vi "Record in xml and EQdb.vi"(8 "error in":errorcluster, 11 "?":T1) -> (0 "error out":errorcluster, 1 "Database primary key":i32, 2 "Variant return data":variant, 3 "Serial number out":string)   [LabVIEW 2018]
uses:
  State data/Records.ctl
  <userlib>/nEQdb/Test Data classes/Basic Data/nEQdb data base enums.ctl
  <userlib>/nEQdb/Test Data classes/Basic Data/Basic Data.lvclass
  C:/Program Files (x86)/National Instruments/LabVIEW 2018/user.lib/nEQdb/Test Data classes/Test Data.lvclass
  <userlib>/nEQdb/Test Data classes/Test Data.lvclass
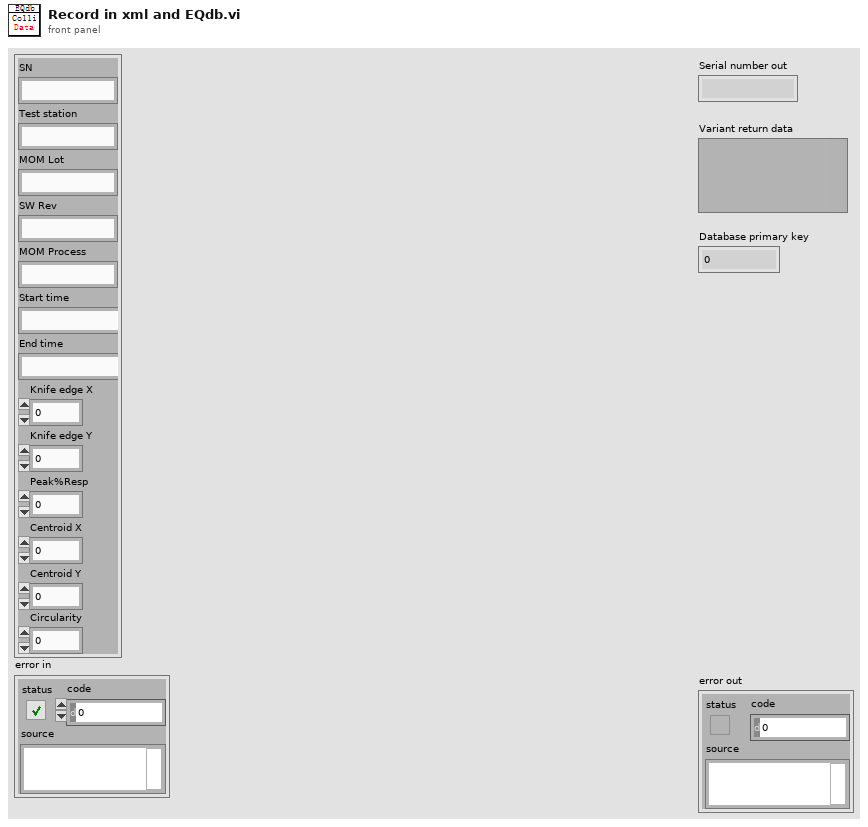
[diagram p1: front panel]
types:
  T1 = typedef "Records.ctl" = cluster{"SN":string, "Test station":string, "MOM Lot":string, "SW Rev":string, "MOM Process":string, "Start time":string, "End time":string, "Knife edge X":dbl, "Peak%Resp":dbl, "Centroid X":dbl, "Knife edge Y":dbl, "Centroid Y":dbl, "Circularity":dbl}
  T2 = typedef "Basic Data.lvclass/nEQdb data base enums.ctl" = enum16{"No enum selected", "Serial number 1", "Test number 2", "Subtest type 3", "Subtest number 4", "Datapoint 5", "Operator 6", "Water temperature supply 7", "Water temperature return 8", "Water pressure supply 9", "Water pressure return 10", "Water flow rate supply 11", "Water flow rate return 12", "Test parameter file 13", "Workorder number 14", "Workorder operation number 15", "Thermal resistance degcperw 16", "Thermal resistance mpera 17", "Current source model 18", "Current source sn 19", "Power meter model 20", "Power meter sn 21", "Power meter head model 22", "Power meter head sn 23", "Threshold current 24", "Slope efficiency 25", "Temperature set 26", "Temperature measured at test start 27", "Power auxilary units 28", "Power auxilary description 29", "Temporary auxilary description 30", "Itar 31", "Dynamic resistance 32", "Voltage intercept 33", "Calibration current 34", "Current set 35", "Current measured 36", "Optical power 37", "Voltage diode 38", "Voltage compliance 39", "Temperature measured 40", "Efficiency diode 41", "Voltage tec 42", "Current tec 43", "Detector responsivity 44", "Detector responsivity wavelength 45", "Power auxilary 46", "Temperature auxilary 47", "Start datetime 48", "End datetime 49", "Centroid 50", "Peak 51", "Fwhm 52", "Fw1 e 2m 53", "Fw1 e 3m 54", "Pulse width 55", "Prf 56", "Osa sensitivity 57", "Osa samples 58", "Osa resolution 59", "Osa averaging 60", "Test station 61", "Additional instruments model 62", "Additional instruments sn 63", "Osa model 64", "Osa sn 65", "Multi stage test key 66", "Good emitters 67", "Wavelength 68", "Intensity 69", "Position 70", "Operating power 71", "Schema 72", "Centroid as pixel 73", "Polarization 74", "Intensity te 75", "Intensity tm 76", "Intensity baseline 77", "Te ratio 78", "Current set scan 79", "Current measured scan 80", "Centroid temporal variation 81", "Voltage 82", "Current 83", "Volt meter model 84", "Volt meter sn 85", "Angle 86", "Farfield axis 87", "Item 88", "Activity 89", "Limit 90", "Operating power spec 91", "Operating current spec 92", "Operating voltage 93", "Operating efficiency 94", "Operating resistance 95", "Reverse bias leakage current 96", "Threshold current change 97", "Slope efficiency change 98", "Operating current change 99", "Active date 100", "Active notes 101", "Eco number 102", "Test notes 103", "Spectral map 104", "Test id from test station 105", "Is image 106", "Image pathname 107", "Datetime 108", "Grade initial 109", "Grade final 110", "Workorder operation name 111", "Engineering grading field 112", "Slope efficiency spec 113", "Threshold current spec 114", "Auxilary identifier 115", "Fwhm fa 116", "Telescope magnification 117", "Measurement lens focal length 118", "Te ratio spec 119", "Wavelength fwhm operating spec 120", "Wavelength fw1e2m operating spec 121", "Prebi slope efficiency spec 122", "Prebi operating current spec 123", "Controlled spec 124", "Wavelength centroid spec 125", "Divergence na 90  incl spec 126", "Wavelength temperature coefficient spec 127", "Operating temperature spec 128", "Fast axis divergence fw1e2m spec 129", "Slow axis divergence fw1e2m spec 130", "Rows of chiplets 131", "Columns of chiplets 132", "Divergence na 90  incl 133", "Fast axis divergence fwhm spec 134", "Slow axis divergence fwhm spec 135", "Farfield current 136", "Nearfield current 137", "Nearfield fwhm 138", "Nearfield fw1e2m 139", "Operating power validation spec 140", "Reverse bias leakage current validation spec 141", "Operating resistance validation spec 142", "Threshold current validation spec 143", "Threshold current change validation spec 144", "Slope efficiency validation spec 145", "Slope efficiency change validation spec 146", "Operating current validation spec 147", "Operating current change validation spec 148", "Te ratio validation spec 149", "Operating efficiency validation spec 150", "Operating voltage validation spec 151", "Thermal resistance degcperw validation spec 152", "Wavelength fwhm validation spec 153", "Wavelength fw1e2m validation spec 154", "Validation wavelength current validation spec 155", "Number of emitters validation spec 156", "Fast axis divergence fwhm validation spec 157", "Slow axis divergence fwhm validation spec 158", "External power supply voltage 159", "Bay 160", "Lens magnification 161", "Scan type 162", "Scan file 163", "Measured optical power 164", "Beam width short axis 165", "Beam length short axis 166", "Beam non uniformity 167", "Beam local non uniformity 168", "Total optical power 169", "Power density 170", "Relative beam position 171", "Subtesttype name 172", "Subtest name 173", "Laser number 174", "System temp label 175", "System flow label 176", "Ldd number 177", "Ldd laser number 178", "Additional instrument description 179", "Micrometer position 180", "Stage position x 181", "Stage position y 182", "Stage position z 183", "Stage position roll 184", "Stage position yaw 185", "Stage position pitch 186", "Mean maximum temperature 187", "Absolute pressure 60s after minimum 188", "Stage position align power 189", "Stage position number 190", "Stage position max align power 191", "Efficiency peak spec 192", "O to o spec 193", "Unit 194", "Qty per series 195", "Qty 196", "Used at operation number 197", "New or already released 198", "Route 199", "Itemname 200", "Recipe name 201", "Maskdatum1 x coord 202", "Maskdatum1 y coord 203", "Maskdatum2 x coord 204", "Maskdatum2 y coord 205", "Layer 206", "Emitter location file pathname 207", "Time 208", "Defect number 209", "X coord 210", "Y coord 211", "Classification 212", "Perimeter straightness 213", "Area width 214", "Brightness 215", "Area diameter 216", "Surface range 217", "Surface range x 218", "Surface range y 219", "Surface gradient 220", "Surface gradient x 221", "Surface gradient y 222", "Maximum gradient x 223", "Area gradient x 224", "Density gradient x 225", "Maximum gradient y 226", "Area gradient y 227", "Density gradient y 228", "Perimeter 229", "Radius mean 230", "Radius minimum mean 231", "Radius maximum mean 232", "Perimeter roundness 233", "Mask region 234", "Centroid x 235", "Centroid y 236", "Enclosing rectangle width 237", "Enclosing rectangle height 238", "Compactness factor 239", "Maximum gradient 240", "Average hue 241", "Hue range 242", "Hue std deviation 243", "Average saturation 244", "Saturation range 245", "Saturation std deviation 246", "Convex hull perimeter 247", "Convex hull area 248", "Convex hull eccentricity 249", "Perimeter eccentricity 250", "Not used at this time  251", "Solidity 252", "Circularity 253", "Orientation 254", "Edge count maximum 255", "Edge count average 256", "Edge count variance 257", "Thin curve length 258", "Thin curve width 259", "Tks power supply configuration 260", "Build number 261", "Component number 262", "Component serial number 263", "Component item number 264", "Pass 265", "Pass fail comment 266", "Pulse energy mean 267", "Pulse energy min 268", "Pulse energy max 269", "Pulse energy stddev 270", "Pulse delay 271", "X divergence mean 272", "X divergence min 273", "X divergence max 274", "X divergence stddev 275", "Y divergence mean 276", "Y divergence min 277", "Y divergence max 278", "Y divergence stddev 279", "Measurement name 280", "Measurement unit 281", "Mean 282", "Min 283", "Max 284", "Stddev 285", "Data reference 286", "Device section 287", "Ccd saturation 288", "Aggregate number 289", "Camera type 290", "Component lot number 291", "Noise equivalent power 292", "Beamview ats pathname 293", "Maximum temperature thermocouple a 294", "Maximum temperature thermocouple b 295", "Maximum temperature thermocouple c 296", "Maximum temperature thermocouple d 297", "Set voltage 298", "Beam rotation 299", "Component position 300", "Build notes 301", "Rmse 302", "Layer thickness 303", "Beamview  knife edge   84  304", "Operation step 305", "Peak responisivity 306", "Tec current to voltage slope 307", "Tec current to voltage intercept 308", "Mpd responsivity 309", "Mpd intercept 310", "Mpd intercept   responsivity 311", "Dark reading 312", "Global wavelength fwhm spec 313", "Global wavelength fw1e2m spec 314", "Liv is monotonically increasing 315", "Fiber temperature 316", "Farfield full na 317", "Farfield partial na 318", "Farfield na ratio 319", "Temperature auxilary 2 description 320", "Temperature auxilary 2 321", "Process step 322", "Min wavelength for pib calc 323", "Max wavelength for pib calc 324", "Power in wavelength band spec 325", "Na aperture transmission spec 326", "Stage position align power delta 327", "Element tpf temperature measuring location 328", "Element tpf operation temp 329", "Element tpf tks current 330", "Element tpf tks pulse duration 331", "Element tpf tks pulse pause 332", "Element tpf mirroring emitter voltage 333", "Element tpf c1 334", "Element tpf c2 335", "Element tpf c3 336", "Element tpf c4 337", "Element tpf c5 338", "Element tpf c6 339", "Element tpf c7 340", "Element tpf c8 341", "Element tpf c9 342", "Element tpf c10 343", "Element tpf c11 344", "Element tpf c12 345", "Element tpf c13 346", "Element tpf c14 347", "Element tpf c15 348", "Element tpf s1 349", "Element tpf s2 350", "Element tpf s3 351", "Element tpf s4 352", "Element tpf s5 353", "Element tpf s6 354", "Element tpf s7 355", "Element tpf s8 356", "Element tpf s9 357", "Element tpf s10 358", "Element calc wave temp shift 359", "Element calc threshold start 360", "Element calc threshold length 361", "Element calc slope start 362", "Element calc slope length 363", "Element calc series resistance start 364", "Element calc series resistance length 365", "Element calc thermal resistance start 366", "Element calc thermal resistance length 367", "Element calc wave shift start 368", "Element calc wave shift length 369", "Element calc iop start 370", "Element calc iop length 371", "Element calc liv graph current max 372", "Element calc liv graph current spacing 373", "Element calc liv graph primary max 374", "Element calc liv graph primary spacing 375", "Element calc liv graph secondary max 376", "Element calc liv graph secondary spacing 377", "Element calc liv graph voltage axis 378", "Element calc liv graph efficiency axis 379", "Element calc spectrum graph min 380", "Element calc spectrum graph max 381", "Min current for pib calc 382", "Max current for pib calc 383", "Operating power change spec 384", "Mom lotid 385", "Mom processid 386", "Mom processstepid 387", "Element tpf bi current 388", "Mom unitid 389", "Mom lotstatushistoryid 390", "Rework designator 391", "Pulse width 90 392", "Pulse rise time 10 90 393", "Pulse fall time 10 90 394", "Pulse width 50 mean 395", "Pulse width 50 min 396", "Pulse width 50 max 397", "Process sub step 398", "Missedpulses 399", "Opticalprf 400", "Pulseenratio 401", "Pulseenmaxproximity 402", "Extratio 403", "Opticalpower 404", "Anglestab 405", "Ffdiv 406", "Angleerror 407", "Nfdiam 408", "Outputloc 409", "Spdoutputcharge w card 410", "Spcca h rise 411", "Spcca l fall 412", "Spcca l high min 413", "Spcca l high max 414", "Spcca l low min 415", "Spcca l low max 416", "Spcca h high min 417", "Spcca h high max 418", "Spcca h low min 419", "Spcca h low max 420", "Firstpulsedelay 421", "Lastpulsedelay 422", "Pulse energy mean   obsolete 423", "Pulse energy min   obsolete 424", "Pulse energy max   obsolete 425", "Currentset1 426", "Currentset2 427", "Power1 428", "Power2 429", "Operating current 430", "Pulse width 50 std dev 431", "Optical prf min 432", "Optical prf max 433", "Optical prf mean 434", "Optical prf std dev 435", "Optical power min 436", "Optical power max 437", "Optical power mean 438", "Optical power std dev 439", "Pulse energy std dev   obsolete 440", "Beam waist  x 441", "Beam waist  y 442", "Beam divergence  x 443", "Beam divergence  y 444", "Waist location  x 445", "Waist location  y 446", "M 2  x 447", "M 2  y 448", "Bpp  x 449", "Bpp  y 450", "Rayleigh range  x 451", "Rayleigh range  y 452", "Astigmatism 453", "Asymmetry 454", "M 2 455", "Jitter  temporal 456", "O to o efficiency 457", "Power  peak 458", "Optical brightness  peak 459", "Boresight  x 460", "Boresight  y 461", "Boresight 462", "Optical pump slope efficiency 463", "Optical pump threshold current 464", "Optical pump wavelength centroid  m 465", "Optical pump wavelength centroid  b 466", "Optical pump power  operating 467", "Optical pump wavelength centroid  operating 468", "Integration time 469", "Fast axis divergence centroid spec 470", "Slow axis divergence centroid spec 471", "Process step for change calculations 472", "Itemid as tested 473", "Horizontal polarization 474", "Vertical polarization 475", "Forward voltage 476", "Angleerror x 477", "Angleerror y 478", "Output loc x 479", "Output loc y 480", "Spdoutputamps w card 481", "Spdwidth w card 482", "Spdrise w card 483", "Stage name 484", "Test type 485", "Measurement number 486", "Operating temperature 487", "Average combiner loss 488", "Cleave angle 489", "Total cleave angle 490", "Splice  power loss 491", "Splice heating rate 492", "Combiner loss 493", "Sensor value 494", "Power aux 2 495", "Power auxilary units 2 496", "Power auxilary description 2 497", "Power aux 3 498", "Power auxilary units 3 499", "Power auxilary description 3 500", "Power aux 4 501", "Power auxilary units 4 502", "Power auxilary description 4 503", "Power aux 5 504", "Power auxilary units 5 505", "Power auxilary description 5 506", "Power aux 6 507", "Power auxilary units 6 508", "Power auxilary description 6 509", "Tbd 510", "Tbd2 511", "Temperature auxilary 3 512", "Temprture aux description 3 513", "Temperature auxilary 4 514", "Temprture aux description 4 515", "Temperature auxilary 5 516", "Temprture aux description 5 517", "Temperature auxilary 6 518", "Temprture aux description 6 519", "Forward bias current spec 520", "Centroid wavelength at hex temp 521", "Centroid wavelength at set hex temp 522", "Configuration file pathname 523", "Min rate of change of slope 524", "Max fw1e2m 525", "Min current for kink calc 526", "Max current for kink calc 527", "Kink size 528", "Max change in fw1e2m 529", "Post solder na 530", "Open gripper na 531", "Initial align na high power 532", "Initial align na low power 533", "Offset to baseline 534", "Align na to baseline 535", "Y position 536", "Na at this y 537", "Divergence na 95  incl spec 538", "Phi rotation 539", "Optical duty factor 540", "Farfield centroid spec 541", "Minimum peak wavelength 542", "Maximum peak wavelength 543", "Centroid wavelength at start of process 544", "Power in band 545", "Power loss 546", "Pulse time 547", "Pulse amplitude 548", "Combiner temperature 1 549", "Duty cycle 550", "Beam dump temperature 551", "Clad light stripper temperature 1 552", "Clad light stripper temperature 2 553", "Clad light stripper temperature 3 554", "Humidity 555", "Ambient temperature 1 556", "Dew point temperature 557", "Water leak 558", "Internal optical power 559", "Clad light stripper photodiode 1a 560", "Clad light stripper photodiode 1b 561", "Clad light stripper photodiode 2a 562", "Clad light stripper photodiode 2b 563", "Beam dump photodiode 564", "Fiber tray photodiode 565", "Combiner in photodiode 566", "Mandrel photodiode 567", "Ambient photodiode 1 568", "Ambient photodiode 2 569", "Splice photodiode 1 570", "Splice photodiode 2 571", "Combiner out photodiode 1 572", "Combiner out photodiode 2 573", "Combiner temperature 2 574", "Ldd temperature 1 575", "Ldd temperature 2 576", "Ldd temperature 3 577", "Ldd temperature 4 578", "Ldd temperature 5 579", "Ldd temperature 6 580", "Ldd temperature 7 581", "Ldd compliance voltage 1 582", "Ambient temperature 2 583", "Fan tach 1 584", "Fan tach 2 585", "Fan tach 3 586", "Fan tach 4 587", "Fan tach 5 588", "Fan tach 6 589", "Fan tach 7 590", "Fan tach 8 591", "Fan tach 9 592", "Fiber end 593", "Distal clad diameter 594", "Distal fiber core diameter 595", "Distal concentricity 596", "Proximal clad diameter 597", "Proximal fiber core diameter 598", "Proximal concentricity 599", "Wavelength centroid 600", "Reflectivity 601", "Slsr 602", "Signal insertion loss 603", "Avg insertion loss pump clad 604", "Total clad loss  best port  605", "Total clad loss  worst port  606", "Total clad loss  avg port  607", "Pump inner clad loss best port 608", "Pump inner clad loss worst port 609", "Pump inner clad loss avg port 610", "Total clad loss p1 611", "Total clad loss p2 612", "Total clad loss p3 613", "Total clad loss p4 614", "Total clad loss p5 615", "Total clad loss p6 616", "Total clad loss p7 617", "Model 618", "Power bin minimum 619", "Power bin range per bin 620", "Power bin number 621", "Super pulse rise time 622", "Warming simmer current 623", "Ldd compliance voltage 2 624", "Ldd compliance voltage 3 625", "Ldd compliance voltage 4 626", "Ldd compliance voltage 5 627", "Ldd compliance voltage 6 628", "Ambient photodiode gain 629", "Clad light stripper temperature 630", "Average gate on delay 631", "Average gate off delay 632", "High voltage 633", "Low voltage 634", "Modulation depth 635", "High fraction 636", "Low fraction 637", "Average pulse amplitude 638", "Power correction factor 639", "Module build xmlid 640", "Concurrent test key 641", "Stddev gate on delay 642", "Peak minus centroid 643", "Software version 644", "Hr active heat rate 645", "Hr fbg heat rate 646", "Active oc heat rate 647", "Oc cls heat rate 648", "Hot spot 1 heat rate 649", "Hot spot 2 heat rate 650", "Hot spot 1 location 651", "Hot spot 2 location 652", "Background temperature 653", "Hr active temperature 654", "Hr fbg temperature 655", "Active oc temperature 656", "Oc cls temperature 657", "Hot spot 1 temperature 658", "Hot spot 2 temperature 659", "Splicer 660", "Enum 661, not used", "Cleaver 662", "Ideal transmission 663", "L cleave angle 664", "R cleave angle 665", "Baseline core signal 666", "Presplice core signal 667", "Postsplice core signal 668", "Splice recovery 669", "Transmission 670", "Manual align x 671", "Manual align y 672", "Manual align counts 673", "Input power 674", "Wavelength at 65a 675", "L fiber angle 676", "R fiber angle 677", "Total fiber angle 678", "Wast location  z 679", "Manual align z 680", "Single pulse amplitude 681", "Offset x 682", "Offset y 683", "Total offset 684", "Active occls heat rate 685", "Oc fbg heat rate 686", "Comb hr heat rate 687", "Hr osc heat rate 688", "Osc oc heat rate 689", "Oc amp heat rate 690", "Amp cls heat rate 691", "Cls bridge heat rate 692", "Srs 693", "Tail 694", "Comb hr splice 808 heat rate 695", "Comb hr splice 808 trans 696", "Comb hr splice 920 heat rate 697", "Comb hr splice 920 trans 698", "Hr active splice 808 heat rate 699", "Hr active splice 808 trans 700", "Hr active splice 920 heat rate 701", "Hr active splice 920 trans 702", "Active oc splice 808 heat rate 703", "Active oc splice 808 trans 704", "Active oc splice 920 heat rate 705", "Active oc splice 920 trans 706", "Oc cls splice 808 heat rate 707", "Oc cls splice 808 trans 708", "Oc cls splice 920 heat rate 709", "Oc cls splice 920 trans 710", "Hr active pre pot heat rate 711", "Hr fbg pre pot heat rate 712", "Active oc pre pot heat rate 713", "Oc cls pre pot heat rate 714", "Hot spot pre pot heat rate 715", "Pre pot cls cleave angle 716", "Comb hr pre splice trans 717", "Comb hr recovery 718", "Comb hr post splice trans 719", "Hr active baseline change 720", "Hr active pre splice trans 721", "Hr active recovery 722", "Hr active post splice trans 723", "Active occls baseline change 724", "Active occls pre splice trans 725", "Active occls recovery 726", "Active occls post splice trans 727", "Testbinname 728", "Testtargetna 729", "Testtargetnatolerance 730", "Enum 731, not used", "Power correction offset 732", "Power before snout adjust 733", "Current before snout adjust 734", "Current after snout adjust 735", "Power after snout adjust 736", "Pump spot size 737", "Pump high power temp slope 738", "Power intercept 739", "Regression coefficient 1 740", "Regression coefficient 2 741", "Pairing process type 742", "Driver analog current low 743", "Driver analog current high 744", "Driver temperature setting low 745", "Driver temperature setting high 746", "Driver anode voltage low 747", "Driver anode voltage high 748", "Driver config analog in min 749", "Driver config analog in max 750", "Driver config current min 751", "Driver config current max 752", "Optimized pump temp 753", "Pump high power temp intercept 754", "Pump low power temp offset 755", "Optimized pump current 756", "Target output power 757", "Target output power config current 758", "Driver config simmer current 759", "Driver config calibration current low set 760", "Driver config calibration current high set 761", "Driver config calibration current high measured 762", "Driver config calibration current low measured 763", "Driver config super pulse on time 764", "Driver config super pulse off time 765", "Driver config fan speed 766", "Driver config pid proportional 767", "Driver config pid integral 768", "Driver config pid derivative 769", "Driver config pid n 770", "Driver config pid integration max 771", "Driver config pid integration min 772", "Driver config pid out max 773", "Driver config pid out min 774", "Nominal beam center x 775", "Nominal beam center y 776", "M 2 focal length 777", "Head beam pointing 778", "Head beam location 779", "Driver config super pulse level 780", "Bex beam waist  x 781", "Bex beam waist  y 782", "Bex beam divergence  x 783", "Bex beam divergence  y 784", "Bex waist location  x 785", "Bex waist location  y 786", "Bex m 2  x 787", "Bex m 2  y 788", "Bex rayleigh range  x 789", "Bex rayleigh range  y 790", "Bex beam diameter location 791", "Bex beam diameter measured 792", "Bex beam pointing 793", "Bex beam location 794", "Bex average power 795", "Resistance measured 796", "Dwell time 797", "Test outcome 798", "Ramp time 799", "Voltage measured 800", "Fw config 801", "Enum 802, not used", "Pre splice l fiber angle 803", "Post splice l fiber angle 804", "Post splice r fiber angle 805", "Pre splice r fiber angle 806", "Pre splice total fiber angle 807", "Post splice total fiber angle 808", "O o slope efficiency 809", "Electrical safety test type 810", "Optical power meter multiplier 811", "Optical power meter offset 812", "Fwhm diameter 813", "Fw1 e 2m diameter 814", "Fw1 e 3m diameter 815", "Centroid diameter 816", "Failure code 817", "Manufacturer 818", "Hardware version 819", "Firmware version 820", "Driver version 821", "Connection 822", "Test setup check sum value 823", "Finland fiber lot number 824", "Maximum insertion loss 825", "Per 826", "Max insertion loss best port 827", "Max insertion loss worst port 828", "Max insertion loss avg port 829", "Maximum insertion loss pump p1 4 830", "Maximum insertion loss pump p2 4 831", "Maximum insertion loss pump p3 4 832", "Pumps fiber lot 833", "Output fiber lot 834", "Signal fiber lot 835", "Pyrometer current 836", "Reflectometer current 837", "Nominal pump wavelength 838", "Nominal output wavelength 839", "Pump optical power 840", "Relativecameraposition 841", "Axis of scan 842", "Ellipticity1 843", "Ellipticity 1 measurement location 844", "Ellipticity 2 845", "Ellipticity 2 measurement location 846", "Slit energy 847", "Bpp 848", "Waist distance 849", "Image distance 850", "Rayleigh range 851", "Collimator focal length 852", "Collimated path length 853", "Set power 854", "Ellipticity near field 855", "Fast axis fw1 e 2m diameter 856", "Slow axis fw1 e 2m diameter 857", "Fast axis pointing 858", "Slow axis pointing 859", "Fast axis beam rotation 860", "Slow axis beam rotation 861", "Pointing offset 862", "High voltage min 863", "High voltage max 864", "High voltage std dev 865", "Srs peak suppression ratio 866", "Signal insertion loss p1 4 867", "Signal insertion loss p2 4 868", "Signal insertion loss p3 4 869", "Output na p1 4 870", "Output na p2 4 871", "Output na p3 4 872", "Supercarrier step height 873", "Station configuration recipeid 874", "Corona setting 875", "Calculated beam waist diameter 876", "Calculated waist distance 877", "Calculated rayleigh distance 878", "Calculated divergence 879", "Object distance 880", "Measured beam waist diameter 881", "Measured waist distance 882", "Measured rayleigh distance 883", "Measured divergence 884", "Beam width 885", "Ellipticity 886", "Edge steepness 887", "Flatness factor 888", "Flatness power 889", "Plateau uniformity 890", "Axial symmetry 891", "Z location 892", "Nf camera peak response 893", "Ff camera peak response 894", "Nf camera exposure 895", "Ff camera exposure 896", "Nf camera pixel size 897", "Ff camera pixel size 898", "Feedingfibersn 899", "Corona motor count 900", "Nf peak response 901", "Enum 902, not used", "Nf pixel size 903", "Ff peak response 904", "Enum 905, not used", "Ff pixel size 906", "Bar median centroid wavelength 907", "Bar mean centroid wavelength 908", "Bar minimum centroid wavelength 909", "Bar maximum centroid wavelength 910", "Wavelength offset 911", "Wavelength bin 912", "Number of emitters in wavelgnth bin 913", "Cleaver 2 914", "Stripper 915", "Proof tester 916", "Epi wafer number 917", "Epi wafer bar number 918", "Numerical aperture 919", "Relative power 920", "Ring number 921", "Relative power in ring 922", "Emitter number 923", "Error code 924", "Error details 925", "Reported power 926", "Analog power control set voltage 927", "Analog power control measured voltage 928", "Pearl testrecipe i1 929", "Pearl testrecipe i2 930", "Pearl testrecipe i3 931", "Pearl testrecipe i4 932", "Pearl testrecipe i5 933", "Pearl testrecipe i6 934", "Pearl testrecipe i7 935", "Pearl testrecipe i8 936", "Pearl testrecipe i9 937", "Pearl testrecipe i10 938", "Pearl testrecipe i11 939", "Pearl testrecipe i12 940", "Pearl testrecipe i13 941", "Pearl testrecipe i14 942", "Nf centroid x position 943", "Nf centroid y position 944", "Ff centroid x position 945", "Ff centroid y position 946", "Calculated na 947", "Relative power for na calculation 948", "Center wavelength 949", "Emitter position 950", "Bar median center wavelength 951", "Bar median peak wavelength 952", "Data ray beam image 953", "Test currents array 954", "Raw detector power reading 955", "Station power factor 956", "Station power offset 957", "Detector power factor 958", "Detector power offset 959", "Cold plate temperature 960", "Package temperature 961", "Ac power total 962", "Ac power factor total 963", "Ac voltage l1 l2 964", "Ac voltage l2 l3 965", "Ac voltage l3 l1 966", "Ac current total 967", "Power bin 968", "Bpp d86 969", "Bpp iso 970", "Calculatedbeamwaistdiameterd86 971", "Calculatedbeamwaistdiameteriso 972", "Calculateddivergenced86 973", "Calculateddivergenceiso 974", "Ac line1 current 975", "Ac line2 current 976", "Ac line3 current 977", "Baseline correction factor 978", "Baseline correction offset 979", "Blast shield factor 980", "Blast shield offset 981", "Element housing temperature offset 982", "Coated pwr 983", "Waste heat 984", "Coated elec eff 985", "Enum 986, not used", "Operating centroid wavelength 987", "Fw1 e 3 at iop 988", "Red 1e3 989", "Max blue fw 1e3 990", "Max red fw 1e3 991", "Efficiency at iop 992", "Voltage at iop 993", "Pib at min spec current 994", "Pib at max spec current 995", "Series resistance 996", "Vbg temp shift c 997", "Vbg temp shift c w 998", "Targetpctthroughaperture 999", "Noapertureopticalsignal 1000", "Aperturedopticalsignal 1001", "Noapertureopticalpower 1002", "Aperturedopticalpower 1003", "Distanceinz 1004", "Aperturediameter 1005", "Targetdiameter 1006", "Actualdiameterx 1007", "Actualdiametery 1008", "Centerx 1009", "Centery 1010", "Startfiberdiameter 1011", "Lefttaperlength 1012", "Waisttaperlength 1013", "Righttaperlength 1014", "Pre heat time 1015", "Taper heat power absolute 1016", "Taper heat power relative 1017", "Taper heat power waist add 1018", "Rotation 1019", "Rotation speed 1020", "Move mode 1021", "Pulling speed 1022", "Sweep motor 1023", "Pre taper tension 1024", "Capillary taper max delta 1025", "Capillary taper diameter 1026", "Capillary taper min 1027", "Capillary taper max 1028", "Taper bundle max delta 1029", "Taper fiber 360 min 1030", "Package cooling liquid 1031", "Power meter water temperature supply 1032", "Power meter water temperature return 1033", "Power meter water pressure supply 1034", "Power meter water pressure return 1035", "Power meter water flow rate supply 1036", "Power meter water flow rate return 1037", "Fiber clamp temperature 1038", "Mom processstepname 1039", "Operating wavelength peak 1040", "Blue 1e3 1041", "Test parameter recipe id 1042", "Test sequence recipe id 1043", "Test aborted 1044", "Corona qr calibration 1045", "Mode scrambler enabled 1046", "Index 0 mode scrambler 1047", "Index 1 mode scrambler 1048", "Index 2 mode scrambler 1049", "Index 3 mode scrambler 1050", "Index 4 mode scrambler 1051", "Index 5 mode scrambler 1052", "Index 6 mode scrambler 1053", "Index 7 mode scrambler 1054", "Index 8 mode scrambler 1055", "Index 9 mode scrambler 1056", "Index 10 mode scrambler 1057", "Index 11 mode scrambler 1058", "Index 12 mode scrambler 1059", "Index 13 mode scrambler 1060", "Index 14 mode scrambler 1061", "Index 15 mode scrambler 1062", "Index 0 max power 1063", "Index 1 max power 1064", "Index 2 max power 1065", "Index 3 max power 1066", "Index 4 max power 1067", "Index 5 max power 1068", "Index 6 max power 1069", "Index 7 max power 1070", "Index 8 max power 1071", "Index 9 max power 1072", "Index 10 max power 1073", "Index 11 max power 1074", "Index 12 max power 1075", "Index 13 max power 1076", "Index 14 max power 1077", "Index 15 max power 1078", "Ffs channel 1079", "Optimization type 1080", "Minimum locked junction temperature 1081", "Maximum locked junction temperature 1082", "Range locked junction temperature 1083", "Process sub step for test global calculations 1084", "Minimum locked junction temperature test global 1085", "Maximum locked junction temperature test global 1086", "Range locked junction temperature test global 1087", "Low power optical feedback 1088", "Fiber combiner input port 1089", "Corona motor index 1090", "Cold locked wavelength 1091", "Analog out 1 measured voltage 1092", "Analog out 2 measured voltage 1093", "Analog out 3 measured voltage 1094", "Analog out 4 measured voltage 1095", "Component column 1096", "Component row 1097", "Fiber height 1098", "Vp3r3amps 1099", "Vp5amps 1100", "Pin11topin13 1101", "Pin4topin6 1102", "Pin20toground 1103", "Pin19toground 1104", "Pin18toground 1105", "Pin17toground 1106", "Pin16toground 1107", "Pin15toground 1108", "Pin14toground 1109", "Pin13toground 1110", "Pin12toground 1111", "Pin11toground 1112", "Pin10toground 1113", "Pin9toground 1114", "Pin8toground 1115", "Pin7toground 1116", "Pin6toground 1117", "Pin5toground 1118", "Pin4toground 1119", "Pin3toground 1120", "Pin2toground 1121", "Pin1toground 1122", "Loggedinuser 1123", "Spcca l prf 1124", "Spcca h prf 1125", "Wcf image 1126", "Measuredwaistposition 1127", "Differencewaistpositions 1128", "Defocusoffiber 1129", "Nominalcentroidx 1130", "Nominalcentroidy 1131", "Calculatedpointing 1132", "Focusshift 1133", "M2degradation 1134", "Pointingchange 1135", "D2 1136", "Beamview  knife edge   84   x 1137", "Beamview  knife edge   84   y 1138", "Ff th 1139", "Ff pd 1140", "Zeros 1141", "Pump th 1142", "Spare1 pd 1143", "Spare1 th 1144", "Spare2 th 1145", "Spare3 th 1146", "Optical monitor pd 1147", "Temp1 th 1148", "Temp2 th 1149", "Temp3 th 1150", "Temp4 th 1151", "Temp5 th 1152", "Temp6 th 1153", "Dcvolts1 vdc 1154", "Dcvolts2 vdc 1155", "Dcvolts3 vdc 1156", "Dcvolts4 vdc 1157", "Dcvolts5 vdc 1158", "Dcvolts6 vdc 1159", "Water out th 1160", "Comb th 1161", "Optical monitor2 pd 1162", "Water in th 1163", "Ps air th 1164", "Amb pump pd 1165", "Bpp pd 1166", "Bpp in pd 1167", "Pcls pd 1168", "Amb comb pd 1169"}
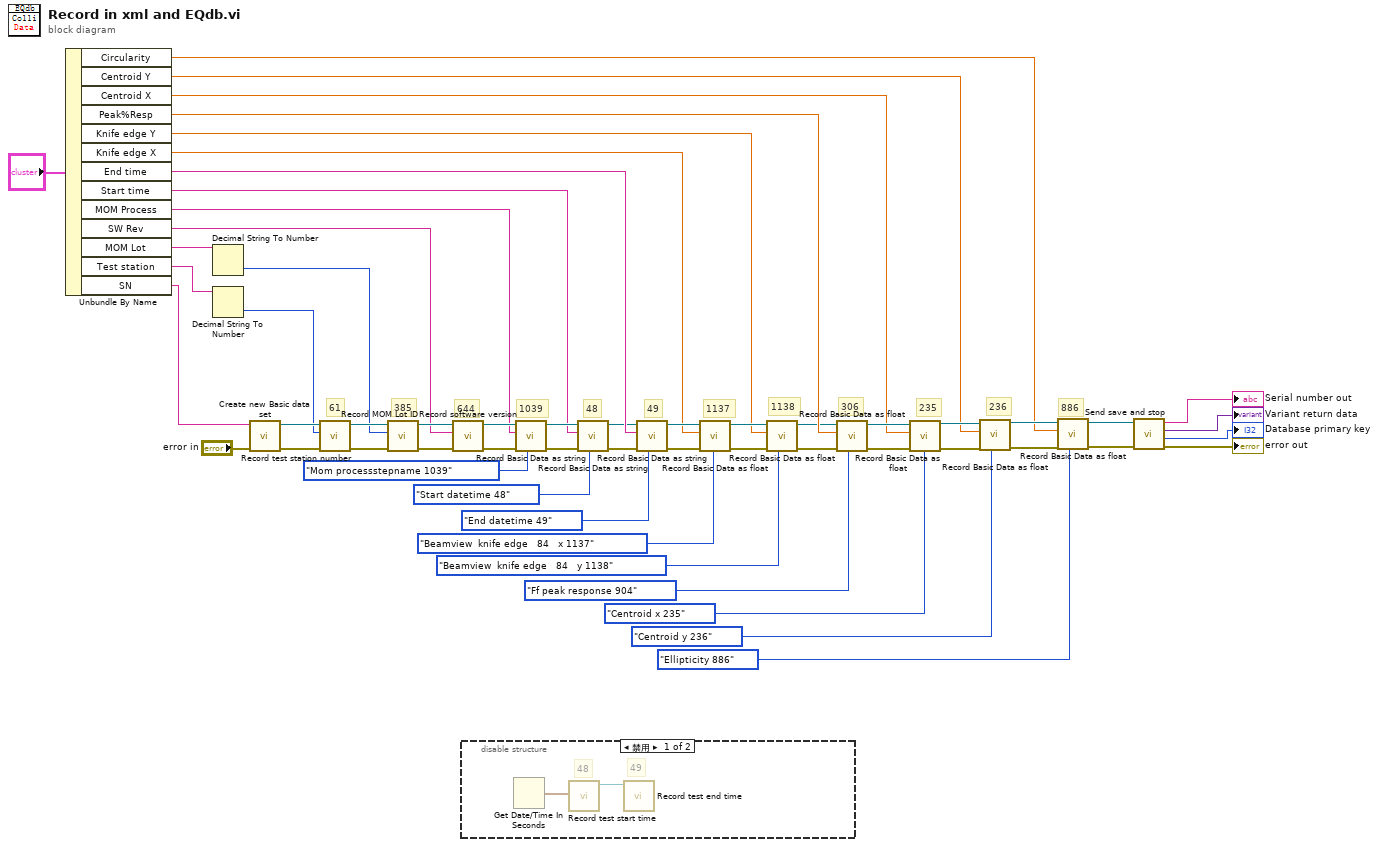
[diagram p0: block diagram]
diagram:
  # "886"
  # "236"
  # "1138"
  # "49"
  # "48"
  # "235"
  # "306"
  # "1137"
  # "1039"
  # "644"
  # "385"
  # "61"
  n1 = Unbundle By Name("?") -> ("Circularity"=w2:dbl, "Centroid Y"=w9:dbl, "Centroid X"=w10:dbl, "Peak%Resp"=w39:dbl, "Knife edge Y"=w11:dbl, "Knife edge X"=w12:dbl, "End time"=w28:string, "Start time"=w27:string, "MOM Process"=w33:string, "SW Rev"=w40:string, "MOM Lot"=w42:string, "Test station"=w38:string, "SN"=w43:string)
  n2 = Decimal String To Number(string=w42) -> (number=w41:i32)  [unwired: 2 in, 1 out]
  n3 = Decimal String To Number(string=w38) -> (number=w37:i32)  [unwired: 2 in, 1 out]
  n4 = call <userlib>:"Create new Basic data set.vi"("error in"="error in", "Serial number"=w43) -> ("error out"=w55:errorcluster, "Basic Data out"=w51:refnum<class "Basic Data.lvclass">)  [unwired: 8 in]
  n5 = call-dynamic "Record test station number.vi"("error in (no error)"=w55, "Test station number"=w37, "Basic Data in"=w51) -> ("error out"=w54:errorcluster, "Basic Data out"=w50:refnum<class "Basic Data.lvclass">)  [unwired: 7 in]
  n6 = call-dynamic "Record MOM Lot ID.vi"("error in (no error)"=w54, "MOM LotID"=w41, "Basic Data in"=w50) -> ("error out"=w53:errorcluster, "Basic Data out"=w49:refnum<class "Basic Data.lvclass">)  [unwired: 7 in]
  n7 = call-dynamic "Record software version.vi"("error in (no error)"=w53, "Software version"=w40, "Basic Data in"=w49) -> ("error out"=w36:errorcluster, "Basic Data out"=w35:refnum<class "Basic Data.lvclass">)  [unwired: 7 in]
  n8 = disable-structure shown="禁用" {
    frame Disabled {
      # "49"
      # "48"
      n9 = Get Date/Time In Seconds() -> (seconds since 1Jan1904=w57:timestamp)
      n10 = call-dynamic "Record test start time.vi"("Start time (Now)"=w57) -> ("Basic Data out"=w58:refnum<class "Basic Data.lvclass">)  [unwired: 9 in, 1 out]
      n11 = call-dynamic "Record test end time.vi"("Basic Data in"=w58) -> ()  [unwired: 9 in, 2 out]
    }
    frame Enabled {
    }
  }
  n12 = call <userlib>:"Record Basic Data as string.vi"("Enum from nEQdb"=nEQdb_data_base_enums."Mom processstepname 1039", "error in (no error)"=w36, "Data as string to record"=w33, "Basic Data in"=w35) -> ("error out"=w32:errorcluster, "Basic Data out"=w31:refnum<class "Basic Data.lvclass">)  [unwired: 6 in]
  n13 = call <userlib>:"Record Basic Data as string.vi"("Enum from nEQdb"=nEQdb_data_base_enums."Start datetime 48", "error in (no error)"=w32, "Data as string to record"=w27, "Basic Data in"=w31) -> ("error out"=w25:errorcluster, "Basic Data out"=w26:refnum<class "Basic Data.lvclass">)  [unwired: 6 in]
  n14 = call <userlib>:"Record Basic Data as string.vi"("Enum from nEQdb"=nEQdb_data_base_enums."End datetime 49", "error in (no error)"=w25, "Data as string to record"=w28, "Basic Data in"=w26) -> ("error out"=w22:errorcluster, "Basic Data out"=w21:refnum<class "Basic Data.lvclass">)  [unwired: 6 in]
  n15 = call <userlib>:"Record Basic Data as float.vi"("Enum from nEQdb"=nEQdb_data_base_enums."Beamview  knife edge   84   x 1137", "error in (no error)"=w22, "Data as floating point to record"=w12, "Basic Data in"=w21) -> ("error out"=w20:errorcluster, "Basic Data out"=w19:refnum<class "Basic Data.lvclass">)  [unwired: 6 in]
  n16 = call <userlib>:"Record Basic Data as float.vi"("Enum from nEQdb"=nEQdb_data_base_enums."Beamview  knife edge   84   y 1138", "error in (no error)"=w20, "Data as floating point to record"=w11, "Basic Data in"=w19) -> ("error out"=w18:errorcluster, "Basic Data out"=w17:refnum<class "Basic Data.lvclass">)  [unwired: 6 in]
  n17 = call <userlib>:"Record Basic Data as float.vi"("Enum from nEQdb"=nEQdb_data_base_enums."Ff peak response 904", "error in (no error)"=w18, "Data as floating point to record"=w39, "Basic Data in"=w17) -> ("error out"=w24:errorcluster, "Basic Data out"=w23:refnum<class "Basic Data.lvclass">)  [unwired: 6 in]
  n18 = call <userlib>:"Record Basic Data as float.vi"("Enum from nEQdb"=nEQdb_data_base_enums."Centroid x 235", "error in (no error)"=w24, "Data as floating point to record"=w10, "Basic Data in"=w23) -> ("error out"=w16:errorcluster, "Basic Data out"=w15:refnum<class "Basic Data.lvclass">)  [unwired: 6 in]
  n19 = call <userlib>:"Record Basic Data as float.vi"("Enum from nEQdb"=nEQdb_data_base_enums."Centroid y 236", "error in (no error)"=w16, "Data as floating point to record"=w9, "Basic Data in"=w15) -> ("error out"=w7:errorcluster, "Basic Data out"=w5:refnum<class "Basic Data.lvclass">)  [unwired: 6 in]
  n20 = call <userlib>:"Record Basic Data as float.vi"("Enum from nEQdb"=nEQdb_data_base_enums."Ellipticity 886", "error in (no error)"=w7, "Data as floating point to record"=w2, "Basic Data in"=w5) -> ("error out"=w6:errorcluster, "Basic Data out"=w4:refnum<class "Basic Data.lvclass">)  [unwired: 6 in]
  n21 = call <userlib>:"Send save and stop.vi"("error in (no error)"=w6, "Test Data in"=w4) -> ("error out"=→"error out":errorcluster, "Database primary key"=→"Database primary key":i32, "Variant return data"=→"Variant return data":variant, "Serial number"=→"Serial number out":string)  [unwired: 6 in]
